vi "Configure Decision Feedback Equalization Tap Optimization.vi"(6 "Eye Width (0.0)":dbl, 8 "error in (no error)":errorcluster, 9 "Max Tap Value (1.0)":dbl=1.0, 10 "Min Tap Value (0.0)":dbl, 11 "VISA resource name":refnum<visa-resource-name>) -> (0 "error out":errorcluster, 3 "VISA resource name out":refnum<visa-resource-name>)   [LabVIEW 2020, in "Agilent 90000 Series.lvlib"]
doc: "Configures the optimization parameters for Feed-Forward Equalization."
uses:
  Agilent 90000 Series.lvlib
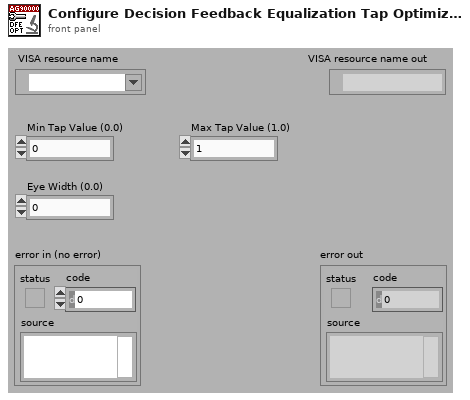
[diagram p1: front panel]
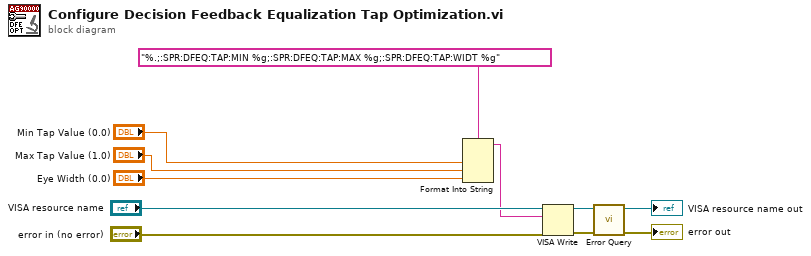
[diagram p0: block diagram]
diagram:
  n1 = Format Into String(format string="%.;:SPR:DFEQ:TAP:MIN %g;:SPR:DFEQ:TAP:MAX %g;:SPR:DFEQ:TAP:WIDT %g", "Min Tap Value (0.0)", "Max Tap Value (1.0)", "Eye Width (0.0)") -> (resulting string=w4:string)  [unwired: 2 in, 1 out]
  n2 = VISA Write(VISA resource name="VISA resource name", write buffer=w4, error in (no error)="error in (no error)") -> (VISA resource name out=w9:refnum<visa-resource-name>, error out=w8:errorcluster)  [unwired: 1 out]
  n3 = call "Error Query.vi"("error in (no error)"=w8, "VISA resource name"=w9) -> ("error out"=→"error out":errorcluster, "VISA resource name out"=→"VISA resource name out":refnum<visa-resource-name>)  [unwired: 8 out]
